vi "Load RampWaveForm from SpreadSheet.vi"(11 "Path":path) -> (3 "RampWaveForms Array":T1[](array[typedef]) {"Waveform"."Start" min=0.0 max=1.0 format="%.2f"; "Waveform"."Time" format="%#_6p"; "Waveform"."End" min=0.0 max=1.0 format="%.2f"})   [LabVIEW 2013]
uses:
  PreciseRampWaveformWithName.ctl
  PreciseRampWaveform.ctl
  <vilib>/Utility/file.llb/Read From Spreadsheet File (string).vi
panel:
  in  "Waveform In":T1={"Name"="", "Waveform"={"Start"=1.0, "End"=256.0, "Time"=1.0}} caption="Cluster" {"Waveform"."Start" min=0.0 max=1.0 format="%.2f"; "Waveform"."End" min=0.0 max=1.0 format="%.2f"}
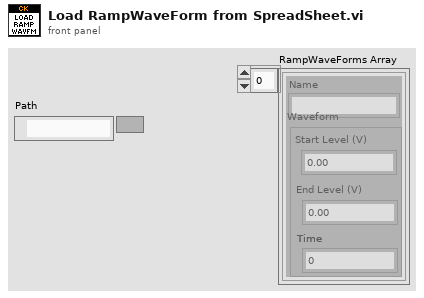
[diagram p1: front panel]
types:
  T1 = typedef "PreciseRampWaveformWithName.ctl" = cluster{"Name":string, "Waveform":T2}
  T2 = typedef "PreciseRampWaveform.ctl" = cluster{"Start":dbl, "End":dbl, "Time":dbl}
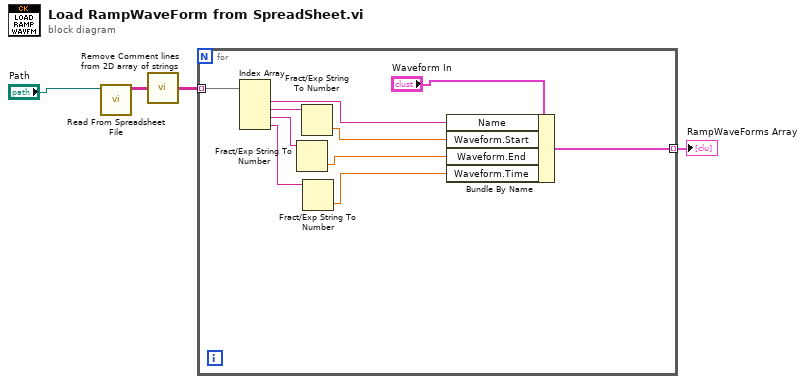
[diagram p0: block diagram]
diagram:
  n1 = call-poly <vilib>:"Read From Spreadsheet File.vi"("file path (dialog if empty)"="Path") -> ("all rows"=w2:string[][])  [unwired: 6 in, 4 out]
  n2 = call "Remove Comment lines from 2D array of strings.vi"("Array in"=w2) -> ("Array out"=w1:string[][])
  n3 = for {
    tunnel: w1 -> [w14] mode=indexing
    tunnel: [w8] -> w3 mode=indexing
    n4 = Index Array(array=w14) -> (element #1=w13:string, element #2=w12:string, element #3=w9:string, element #4=w5:string)  [unwired: 4 in]
    n5 = Fract/Exp String To Number(string=w9) -> (number=w10:dbl)  [unwired: 3 in, 1 out]
    n6 = Fract/Exp String To Number(string=w12) -> (number=w11:dbl)  [unwired: 3 in, 1 out]
    n7 = Fract/Exp String To Number(string=w5) -> (number=w6:dbl)  [unwired: 3 in, 1 out]
    n8 = Bundle By Name(cluster="Waveform In", "Name"=w13, "Waveform.Start"=w11, "Waveform.End"=w10, "Waveform.Time"=w6) -> (w8:T1)
  }
  "RampWaveForms Array" <- w3
